vi "IC_GPOut.vi"(1 "GPOut Value":dbl, 2 "ICImagingControl 3":refnum<k7>) -> (0 "ICImagingControl 2":refnum<k7>)   [LabVIEW 2010]
doc: "Set the GP Out state of a camera."
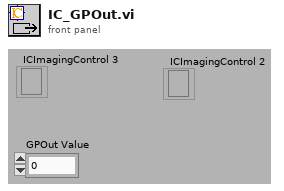
[diagram p1: front panel]
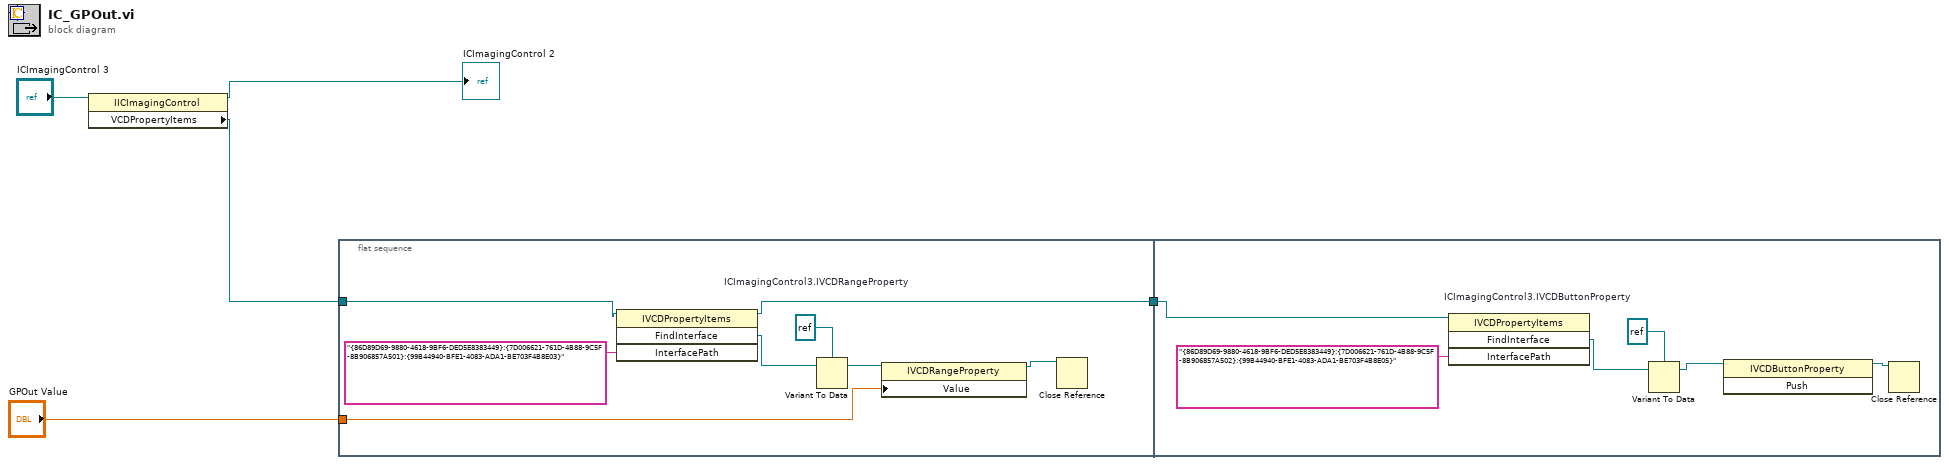
[diagram p0: block diagram]
diagram:
  n1 = property class="IICImagingControl"(reference="ICImagingControl 3") -> (reference out=→"ICImagingControl 2":refnum<k7>, "VCDPropertyItems"=w4:refnum<k7>)  [unwired: 1 in, 1 out]
  n2 = flat-sequence {
    tunnel: w4 -> [w11]
    tunnel: [w10] -> w2
    tunnel: "GPOut Value" -> [w6]
    tunnel: w2 -> [w14]
    frame #0 {
      w9 = refnum<k7> refnum  # ICImagingControl3.IVCDRangeProperty
      n3 = invoke class="IVCDPropertyItems" method="FindInterface"(reference=w11, "InterfacePath"="{86D89D69-9880-4618-9BF6-DED5E8383449}:{7D006621-761D-4B88-9C5F-8B906857A501}:{99B44940-BFE1-4083-ADA1-BE703F4B8E03}") -> (reference out=w10:refnum<k7>, "FindInterface"=w12:refnum<k7>)  [unwired: 2 in, 2 out]
      n4 = Variant To Data(Variant=w12, type=w9) -> (data=w8:refnum<k7>)  [unwired: 1 in, 1 out]
      n5 = property class="IVCDRangeProperty"(reference=w8, "Value"=w6) -> (reference out=w7:refnum<k7>)  [unwired: 1 in, 1 out]
      n6 = Close Reference(reference=w7) -> ()  [unwired: 1 in, 1 out]
    }
    frame #1 {
      w17 = refnum<k7> refnum  # ICImagingControl3.IVCDButtonProperty
      n7 = invoke class="IVCDPropertyItems" method="FindInterface"(reference=w14, "InterfacePath"="{86D89D69-9880-4618-9BF6-DED5E8383449}:{7D006621-761D-4B88-9C5F-8B906857A502}:{99B44940-BFE1-4083-ADA1-BE703F4B8E05}") -> ("FindInterface"=w18:refnum<k7>)  [unwired: 2 in, 3 out]
      n8 = Variant To Data(Variant=w18, type=w17) -> (data=w16:refnum<k7>)  [unwired: 1 in, 1 out]
      n9 = invoke class="IVCDButtonProperty" method="Push"(reference=w16) -> (reference out=w15:refnum<k7>)  [unwired: 2 in, 2 out]
      n10 = Close Reference(reference=w15) -> ()  [unwired: 1 in, 1 out]
    }
  }
